vi "test_gwintek.vi"() -> ()   [LabVIEW 2018]
uses:
  Downloads/LVdriver_AFG-2225_V1_E/AFG-2225/AFG-2225.lvlib
panel:
  in  "Serial Configuration":T1={"Baud Rate"=9600, "Parity"=0, "Data Bits"=8} {"Data Bits" items=["7"=7, "8"=8]; "Parity" items=["None", "Odd", "Even", "Mark", "Space"]; "Baud Rate" items=["300"=300, "600"=600, "1200"=1200, "2400"=2400, "4800"=4800, "9600"=9600, "19200"=19200]}
  in  "Channel":u16(ring) items=["CH1", "CH2"]
  in  "DC Offset (0.00 V)":dbl
  in  "Frequency (1000 Hz)":dbl=1000.0
  in  "Amplitude (0.1 Vpp)":dbl=0.1
  in  "Waveform Function (0: Sine)":u16(ring) items=["Sine", "Square", "Triangle"]
  in  "VISA resource name":refnum<visa-resource-name>
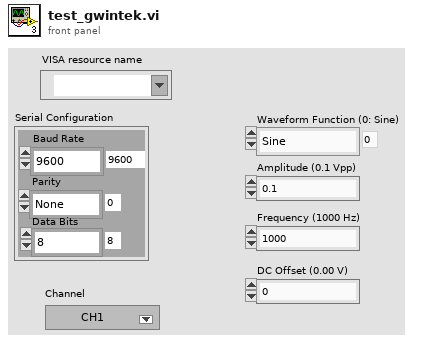
[diagram p1: front panel]
types:
  T1 = cluster{"Baud Rate":u32, "Parity":u16, "Data Bits":u16}
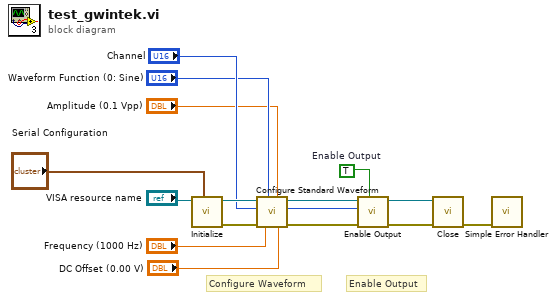
[diagram p0: block diagram]
diagram:
  w9 = TRUE  # Enable Output
  # "Enable Output"
  # "Configure Waveform"
  n1 = call "Initialize.vi"("Serial Configuration"="Serial Configuration", "VISA resource name"="VISA resource name") -> ("error out"=w14:errorcluster, "VISA resource name out"=w15:refnum<visa-resource-name>)  [unwired: 3 in, 5 out]
  n2 = call "Configure Standard Waveform.vi"("DC Offset (0.00 V)"="DC Offset (0.00 V)", "Amplitude (3.000 Vpp)"="Amplitude (0.1 Vpp)", "Frequency (1000.000 Hz)"="Frequency (1000 Hz)", "Waveform Function (0: Sine)"="Waveform Function (0: Sine)", "error in (no error)"=w14, "Channel (0: CH1)"="Channel", "VISA resource name"=w15) -> ("error out"=w8:errorcluster, "Channel out"=w7:u16, "VISA resource name out"=w12:refnum<visa-resource-name>)  [unwired: 1 in, 1 out]
  n3 = call "Enable Output.vi"("Enable Output (T: Enable)"=w9, "error in (no error)"=w8, "Channel (0: CH1)"=w7, "VISA resource name"=w12) -> ("error out"=w10:errorcluster, "VISA resource name out"=w11:refnum<visa-resource-name>)  [unwired: 6 out]
  n4 = call "Close.vi"("error in (no error)"=w10, "VISA resource name"=w11) -> ("error out"=w13:errorcluster)  [unwired: 9 out]
  n5 = call <vilib>:"Simple Error Handler.vi"("error in (no error)"=w13) -> ()  [unwired: 1 in, 8 out]
